vi "SLSC Convert Items - String to Variants.vi"(0 "Datatype":string, 5 "Value":string, 9 "Reset Value":string, 12 "enums":T1[](array[typedef]), 13 "string enums":cluster{"name":string, "string enums":string}[](array[cluster])) -> (4 "Value":variant, 6 "Reset Value":variant, 8 "Value (DBL)":dbl, 10 "Reset Value (DBL)":dbl)   [LabVIEW 2017, in "SLSC Tree Control.lvlib"]
doc: "Converts the string values of the tree control to variants and doubles datatypes."
uses:
  SLSC Tree Control.lvlib
  SLSC EDS API/JSON parsing/enum.ctl
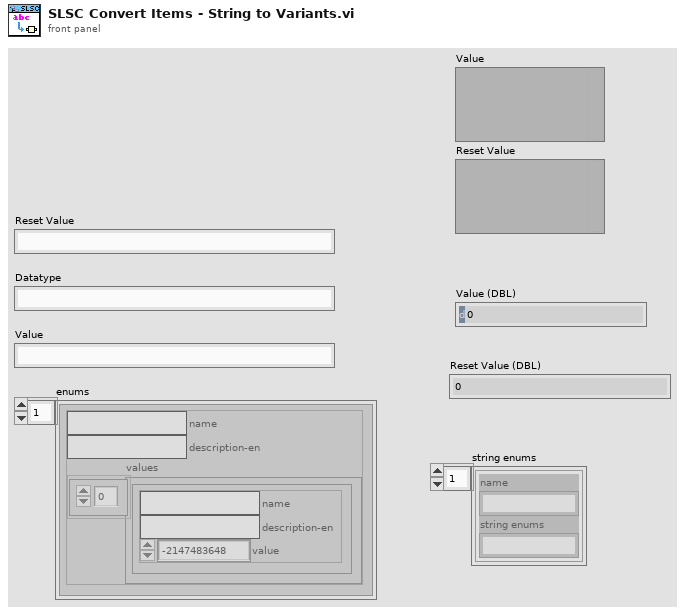
[diagram p1: front panel]
types:
  T1 = typedef "enum.ctl" = cluster{"name":string, "description-en":string, "values":cluster{"name":string, "description-en":string, "value":i32}[]}
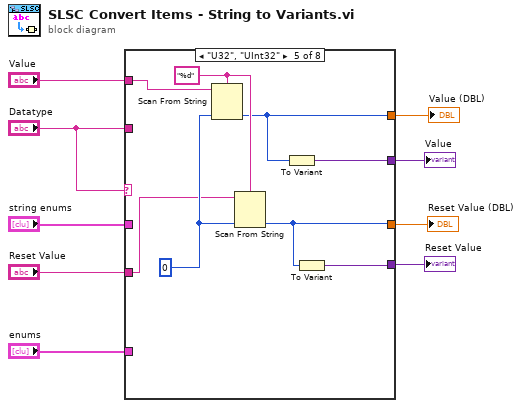
[diagram p0: block diagram]
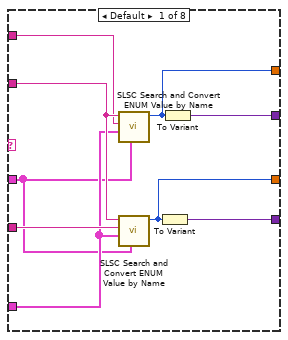
[diagram p2: hidden frame]
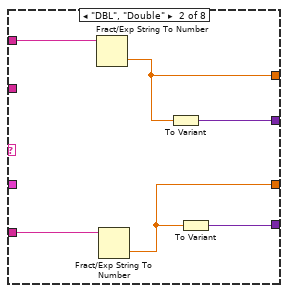
[diagram p3: hidden frame]
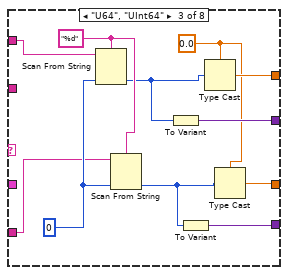
[diagram p4: hidden frame]
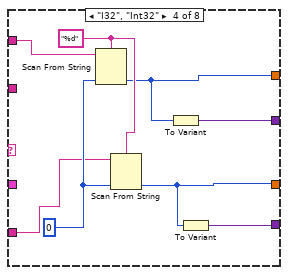
[diagram p5: hidden frame]
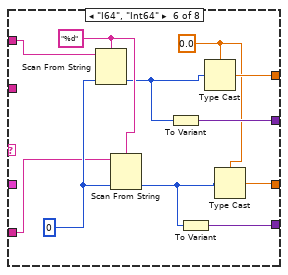
[diagram p6: hidden frame]
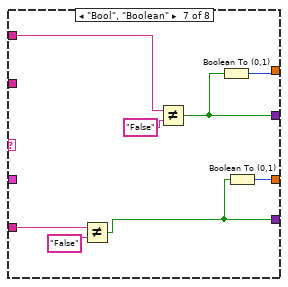
[diagram p7: hidden frame]
diagram:
  n1 = case shown="\"U32\", \"UInt32\"" "Datatype" {
    tunnel: "Reset Value" -> [w18 w22 w31 w40 w47 w58 w68 _]
    tunnel: "Datatype" -> [w17 _ _ _ _ _ _ _]
    tunnel: "enums" -> [w16 _ _ _ _ _ _ _]
    tunnel: "string enums" -> [w15 _ _ _ _ _ _ _]
    tunnel: "Value" -> [w14 w23 w33 w36 w49 w60 w67 w71]
    tunnel: [w13 w24 w35 w43 w51 w62 w65 w71] -> w4
    tunnel: [w12 w21 w34 w42 w50 w61 w63 _] -> w3
    tunnel: [w11 w20 w28 w38 w45 w55 w66 _] -> w2
    tunnel: [w10 w19 w27 w37 w44 w54 w64 _] -> w1
    frame Default {
      n2 = call "SLSC Search and Convert ENUM Value by Name.vi"("Enum Strings"=w15, "enums"=w16, "Value"=w14, "Datatype Name"=w17) -> ("Value"=w11:i32)  [unwired: 5 in, 2 out]
      n3 = call "SLSC Search and Convert ENUM Value by Name.vi"("Enum Strings"=w15, "enums"=w16, "Value"=w18, "Datatype Name"=w17) -> ("Value"=w10:i32)  [unwired: 5 in, 2 out]
      n4 = To Variant(anything=w10) -> (Variant=w12:variant)
      n5 = To Variant(anything=w11) -> (Variant=w13:variant)
    }
    frame "DBL", "Double" {
      n6 = Fract/Exp String To Number(string=w23) -> (number=w20:dbl)  [unwired: 3 in, 1 out]
      n7 = Fract/Exp String To Number(string=w22) -> (number=w19:dbl)  [unwired: 3 in, 1 out]
      n8 = To Variant(anything=w20) -> (Variant=w24:variant)
      n9 = To Variant(anything=w19) -> (Variant=w21:variant)
    }
    frame "U64", "UInt64" {
      w25 = 0.0 ("Value")
      w30 = "%d" ("format string")
      w32 = u64 0 ("default (0 U32)")
      n10 = Scan From String(format string=w30, input string=w33, default 1=w32) -> (output 1=w29:u64)  [unwired: 2 in, 3 out]
      n11 = Scan From String(format string=w30, input string=w31, default 1=w32) -> (output 1=w26:u64)  [unwired: 2 in, 3 out]
      n12 = To Variant(anything=w29) -> (Variant=w35:variant)
      n13 = To Variant(anything=w26) -> (Variant=w34:variant)
      n14 = Type Cast(type=w25, x=w29) -> (*(type *) &x=w28:dbl)
      n15 = Type Cast(type=w25, x=w26) -> (*(type *) &x=w27:dbl)
    }
    frame "I32", "Int32" {
      w39 = "%d" ("format string")
      w41 = 0 ("default (0 U32)")
      n16 = Scan From String(format string=w39, input string=w36, default 1=w41) -> (output 1=w38:i32)  [unwired: 2 in, 3 out]
      n17 = Scan From String(format string=w39, input string=w40, default 1=w41) -> (output 1=w37:i32)  [unwired: 2 in, 3 out]
      n18 = To Variant(anything=w38) -> (Variant=w43:variant)
      n19 = To Variant(anything=w37) -> (Variant=w42:variant)
    }
    frame "U32", "UInt32" {
      w46 = "%d" ("format string")
      w48 = u32 0 ("default (0 U32)")
      n20 = Scan From String(format string=w46, input string=w49, default 1=w48) -> (output 1=w45:u32)  [unwired: 2 in, 3 out]
      n21 = Scan From String(format string=w46, input string=w47, default 1=w48) -> (output 1=w44:u32)  [unwired: 2 in, 3 out]
      n22 = To Variant(anything=w45) -> (Variant=w51:variant)
      n23 = To Variant(anything=w44) -> (Variant=w50:variant)
    }
    frame "I64", "Int64" {
      w52 = 0.0 ("Value")
      w57 = "%d" ("format string")
      w59 = i64 0 ("default (0 U32)")
      n24 = Scan From String(format string=w57, input string=w60, default 1=w59) -> (output 1=w56:i64)  [unwired: 2 in, 3 out]
      n25 = Scan From String(format string=w57, input string=w58, default 1=w59) -> (output 1=w53:i64)  [unwired: 2 in, 3 out]
      n26 = To Variant(anything=w56) -> (Variant=w62:variant)
      n27 = To Variant(anything=w53) -> (Variant=w61:variant)
      n28 = Type Cast(type=w52, x=w56) -> (*(type *) &x=w55:dbl)
      n29 = Type Cast(type=w52, x=w53) -> (*(type *) &x=w54:dbl)
    }
    frame "Bool", "Boolean" {
      n30 = Not Equal?(x=w68, y="False") -> (x != y?=w63:bool)
      n31 = Not Equal?(x=w67, y="False") -> (x != y?=w65:bool)
      n32 = Boolean To (0,1)(Boolean=w65) -> (0, 1=w66:i16)
      n33 = Boolean To (0,1)(Boolean=w63) -> (0, 1=w64:i16)
    }
    frame "String" {
    }
  }
  "Value" <- w4
  "Reset Value" <- w3
  "Value (DBL)" <- w2
  "Reset Value (DBL)" <- w1
